vi "Untitled 6.vi"() -> ()   [LabVIEW 2011]
uses:
  <vilib>/Utility/file.llb/Read From Spreadsheet File (string).vi
  <vilib>/measure/maspectr.llb/FFT Spectrum (Mag-Phase).vi
  <vilib>/Waveform/WDTOps.llb/WDT Index Channel DBL.vi
  <vilib>/express/express analysis/Spectral/Block/exnSpectralBlock spectral measurements RMS poly.vi
  <vilib>/express/express analysis/Spectral/Block/exnSpectralBlock spectral measurements RMS DDT.vi
  <vilib>/express/express analysis/Spectral/XNode/ExpressSpectralMeasurementsBlockNode.xnode
  <vilib>/measure/NI_MAPro.lvlib
panel:
  out "FFT - (RMS)":dynamicdata(graph)
  out "Waveform Graph":cluster{"f0":dbl, "df":dbl, "magnitude":dbl[]}(graph)
  out "Y fft accel 2":dbl[](graph)
  out "Array":u32[][](array[numeric])
  out "number 2":dbl[](array[numeric])
  out "Y fft accel":dbl[](graph)
  in  "Select Data to Analyse":u16(ring) items=["Data 0", "Data 1"]
  in  "Load in CSV File Data1":path
  out "Data Selected 3":u16
  out "Data Selected 2":u16
  in  "Load in CSV File Data0":path
  out "CSV File":string[][](array[string])
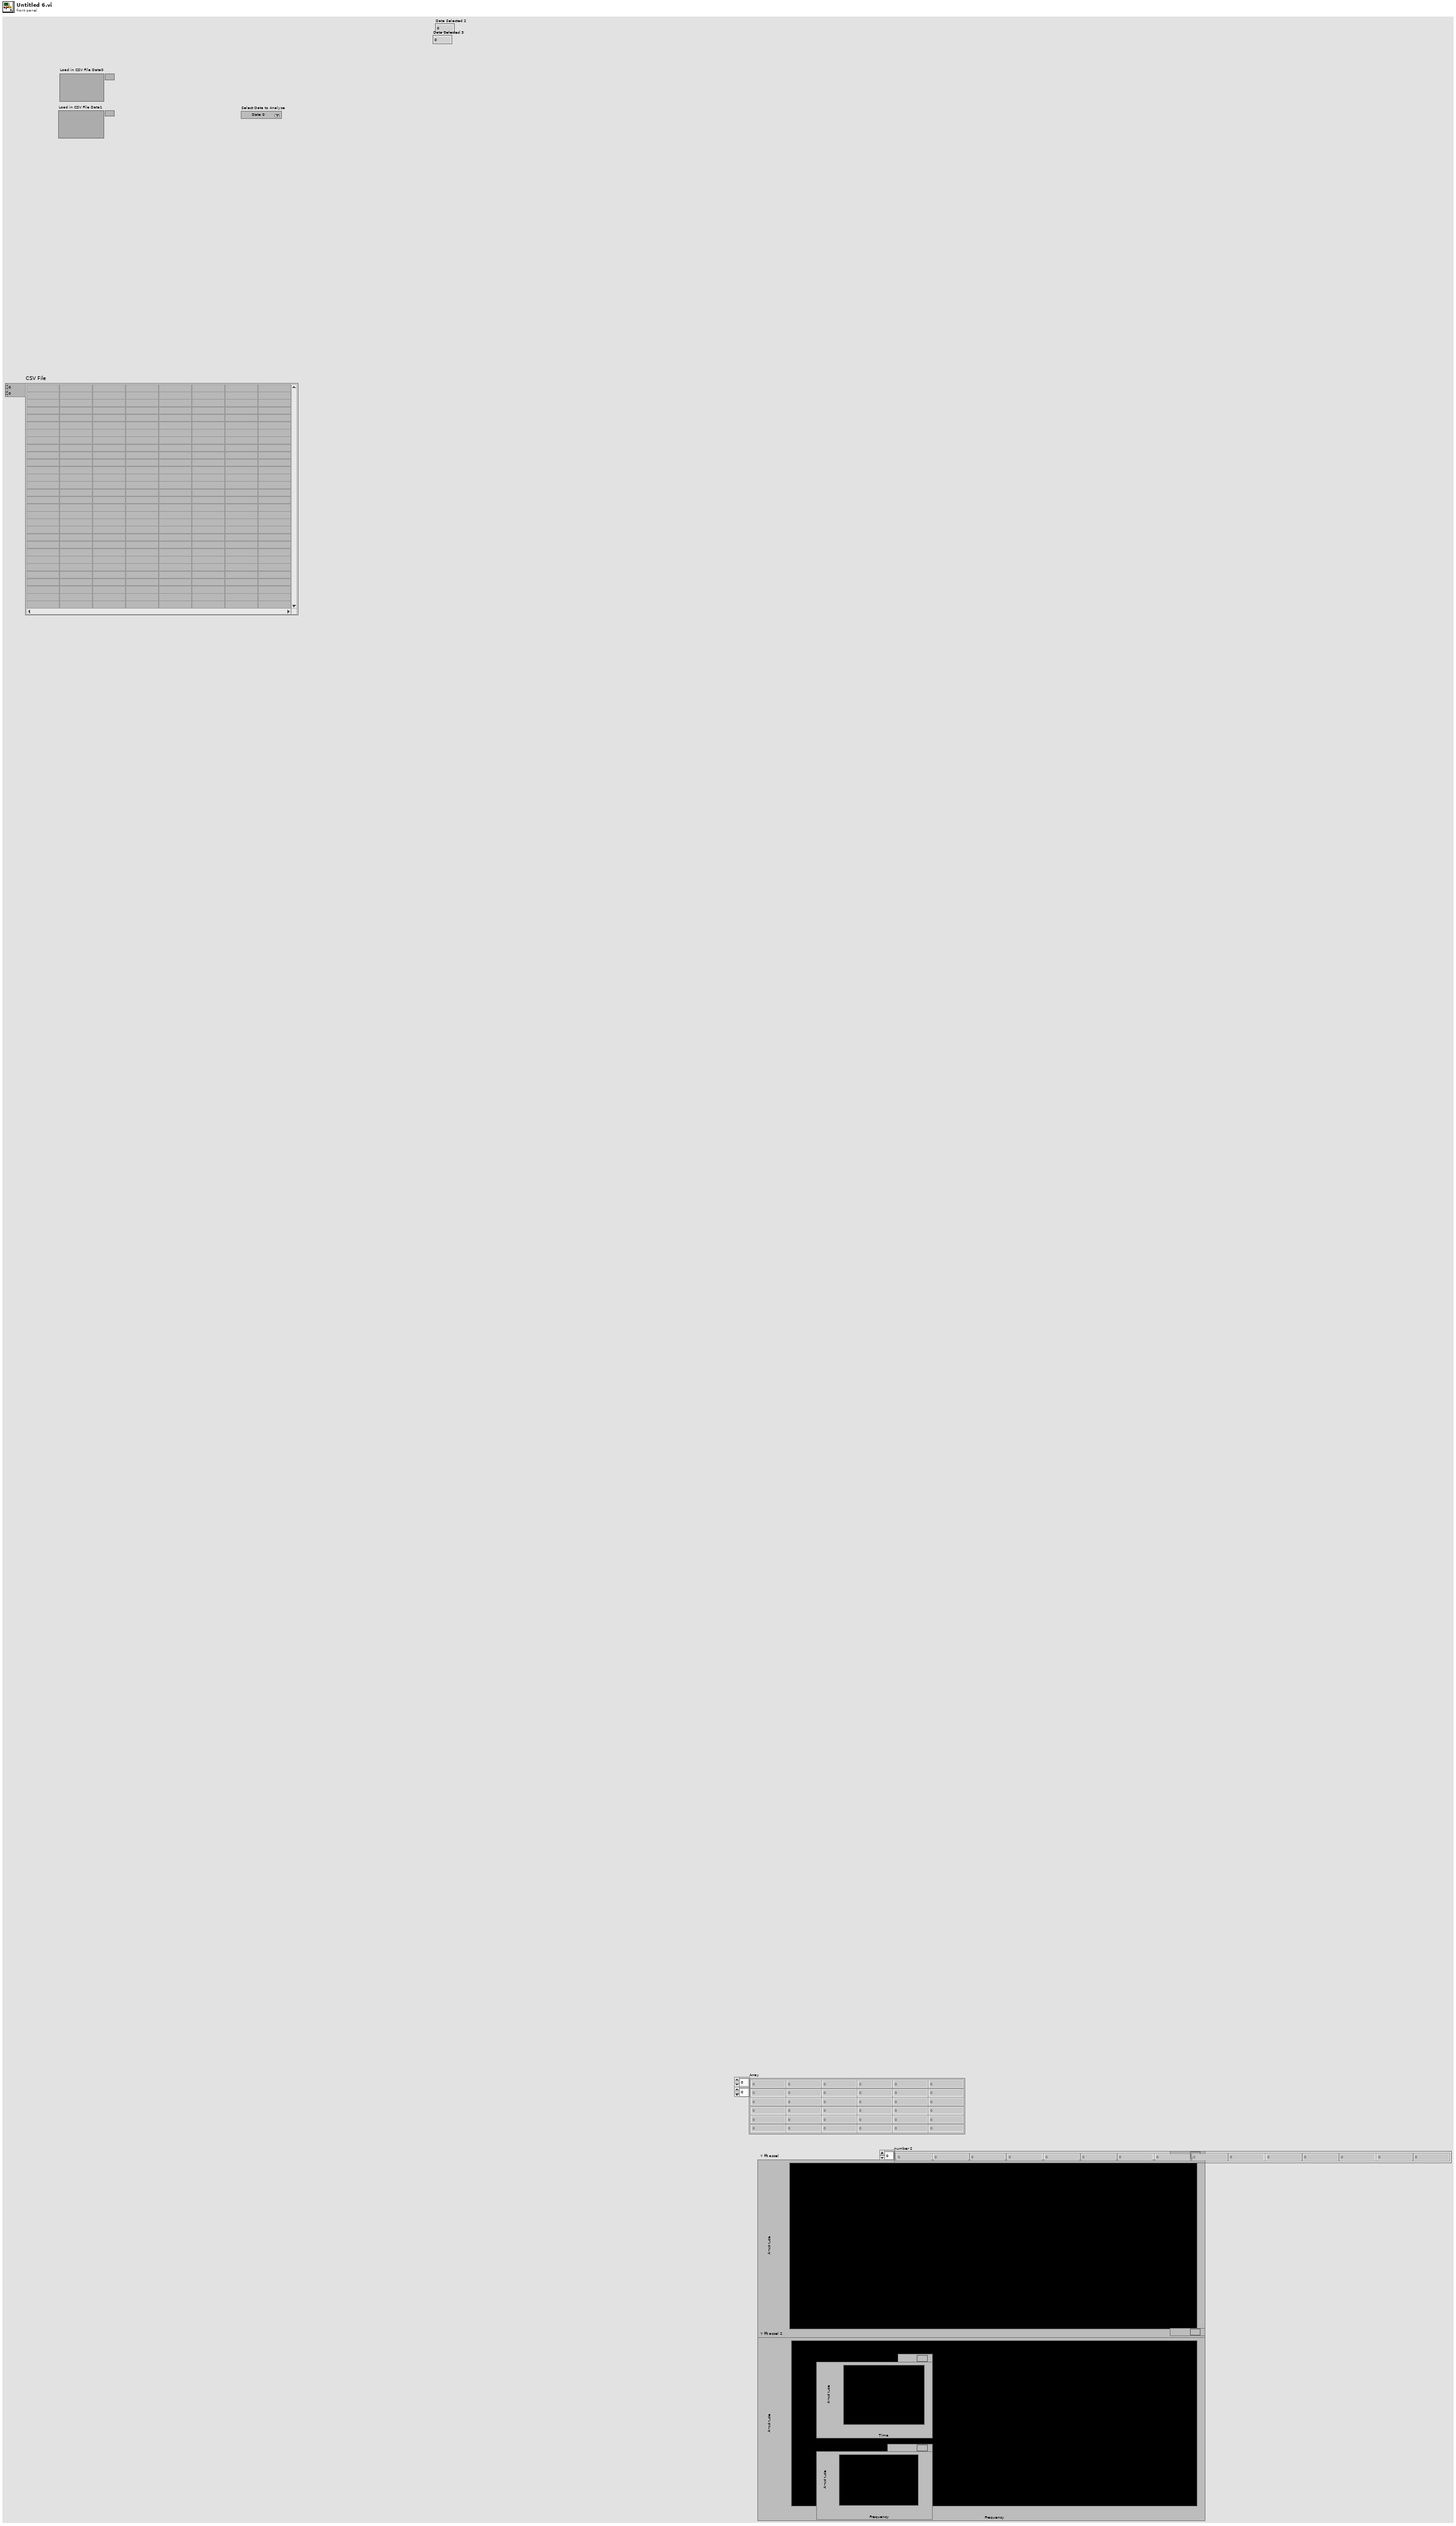
[diagram p1: front panel]
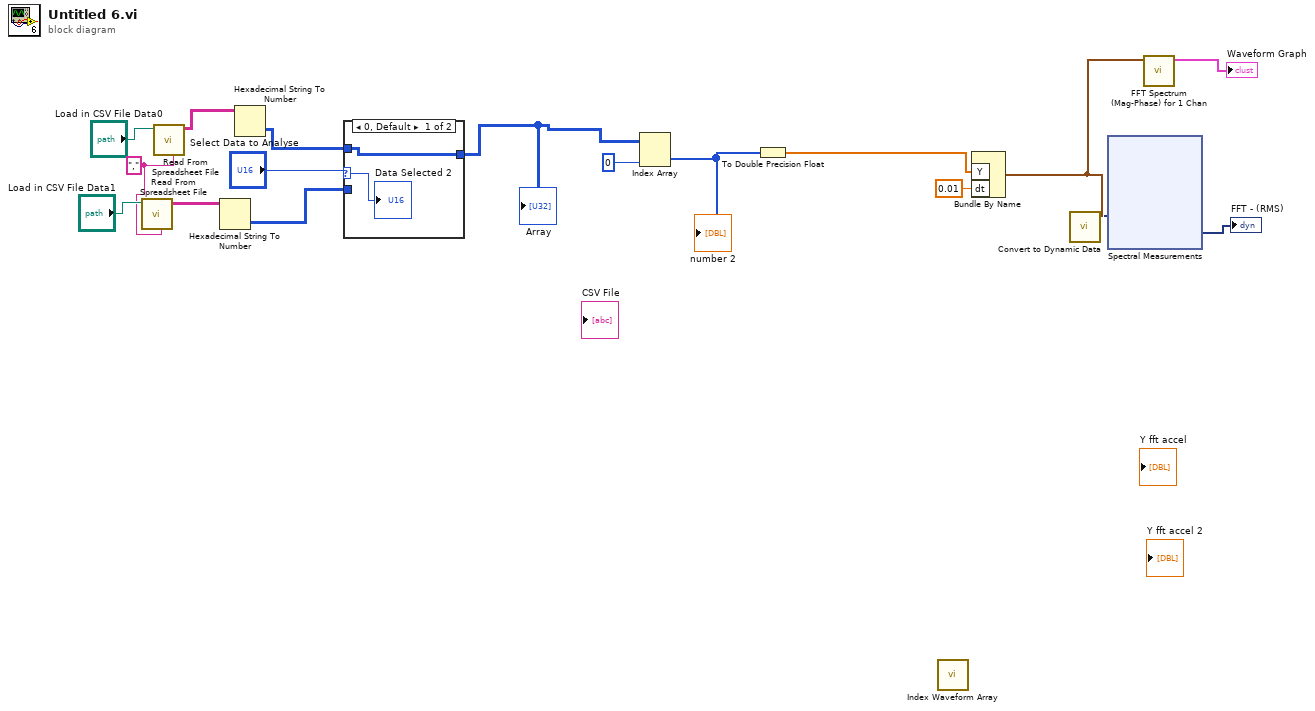
[diagram p0: block diagram]
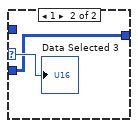
[diagram p2: hidden frame]
diagram:
  w13 = "," ("delimiter (\\t)")
  n1 = call-poly <vilib>:"Read From Spreadsheet File.vi"("delimiter (\\t)"=w13, "file path (dialog if empty)"="Load in CSV File Data1") -> ("all rows"=w14:string[][])  [unwired: 5 in, 4 out]
  n2 = call-poly <vilib>:"Read From Spreadsheet File.vi"("delimiter (\\t)"=w13, "file path (dialog if empty)"="Load in CSV File Data0") -> ("all rows"=w12:string[][])  [unwired: 5 in, 4 out]
  n3 = Hexadecimal String To Number(string=w14) -> (number=w11:u32[][])  [unwired: 2 in, 1 out]
  n4 = Hexadecimal String To Number(string=w12) -> (number=w10:u32[][])  [unwired: 2 in, 1 out]
  n5 = case shown="0, Default" "Select Data to Analyse" {
    selector: "Select Data to Analyse" -> [w19 w21]
    tunnel: w11 -> [_ w20]
    tunnel: [w18 w20] -> w9
    tunnel: w10 -> [w18 _]
    frame 0, Default {
      "Data Selected 2" <- w19
    }
    frame 1 {
      "Data Selected 3" <- w21
    }
  }
  "Array" <- w9
  n6 = Index Array(array=w9, index (col)=0 ("disabled index (col)")) -> (element=w7:u32[])  [unwired: 1 in]
  "number 2" <- w7
  n7 = To Double Precision Float(number=w7) -> (double precision float=w2:dbl[])
  n8 = call-poly <vilib>:"Index Waveform Array.vi"() -> ()  [unwired: 10 in, 2 out]
  n9 = Bundle By Name("Y"=w2, "dt"=0.01) -> (w4:waveform(dbl))  [unwired: 1 in]
  n10 = call "Convert to Dynamic Data"("Waveform"=w4) -> ("Dynamic Data Type"=w3:dynamicdata)  [unwired: 3 in]
  n11 = xnode "Spectral Measurements"("Signals"=w3) -> ("FFT - (RMS)"=→"FFT - (RMS)":dynamicdata)  [unwired: 1 in, 2 out]
  n12 = call-poly <vilib>:"FFT Spectrum (Mag-Phase) for 1 Chan.vi"("time signal"=w4) -> ("magnitude"=→"Waveform Graph":cluster{"f0":dbl, "df":dbl, "magnitude":dbl[]})  [unwired: 6 in, 4 out]
